vi "CreateFilePathDate_Number_Target.vi"(8 "base filename":string, 9 "file number":i32, 10 "Target ID":string, 11 "data filepath":path) -> (3 "appended path":path)   [LabVIEW 2024]
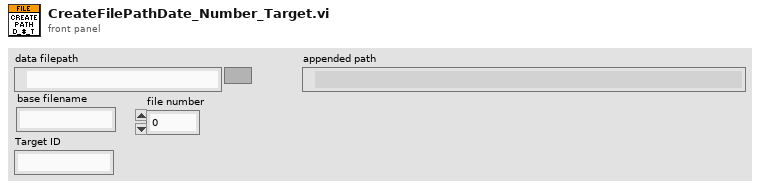
[diagram p1: front panel]
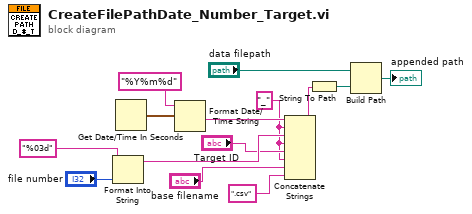
[diagram p0: block diagram]
diagram:
  w3 = "_" ("string")
  n1 = Format Into String(format string="%03d", "file number") -> (resulting string=w5:string)  [unwired: 2 in, 1 out]
  n2 = Get Date/Time In Seconds() -> (seconds since 1Jan1904=w10:timestamp)
  n3 = Format Date/Time String(time format string (%c)="%Y%m%d", seconds (now)=w10) -> (date/time string=w8:string)  [unwired: 1 in]
  n4 = Concatenate Strings(w8, w3, w5, w3, "Target ID", w3, "base filename", ".csv" ("string")) -> (w11:string)
  n5 = String To Path(string=w11) -> (path=w13:path)
  n6 = Build Path(base path="data filepath", name or relative path=w13) -> (appended path=→"appended path":path)
